vi "Read Channel info.vi"(8 "error in":errorcluster, 11 "channel in":refnum<class "StepNode.lvclass">) -> (0 "error out":errorcluster, 2 "channel info":T1, 3 "channel out":refnum<class "StepNode.lvclass">)   [LabVIEW 2015]
doc: "Copyright 2017 National Instruments Corporation\n\nLicensed under the Apache License, Version 2.0 (the \"License\"); you may not use this file except in compliance with the License. You may obtain a copy of the License at http://www.apache.org/licenses/LICENSE-2.0\nUnless required by applicable law or agreed to in writing, software distributed under the License is distributed on an \"AS IS\" BASIS, WITHOUT WARRANTIES OR CONDITIONS OF ANY KIND, either express or implied. See the License for the specific language governing permissions and limitations under the License."
uses:
  StepNode.lvclass
  to delete/ChannelData.ctl
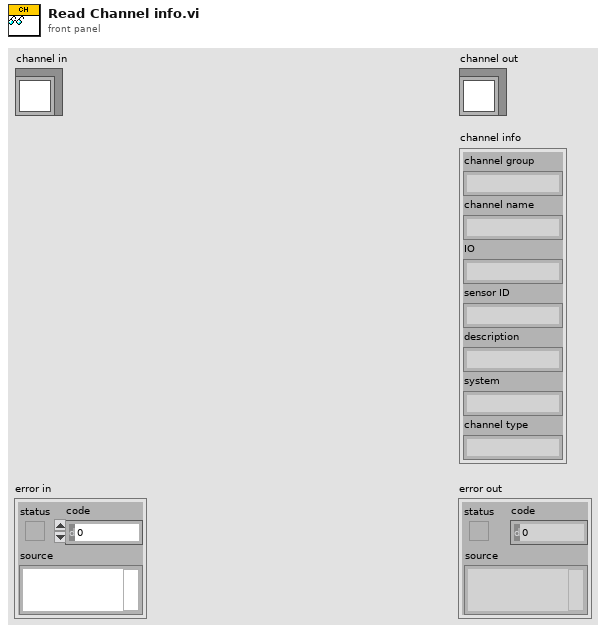
[diagram p1: front panel]
types:
  T1 = typedef "SequenceRepo.lvclass/ChannelData.ctl" = cluster{"channel group":string, "channel name":string, "IO ":string, "sensor ID":string, "description":string, "system":string, "channel type":string}
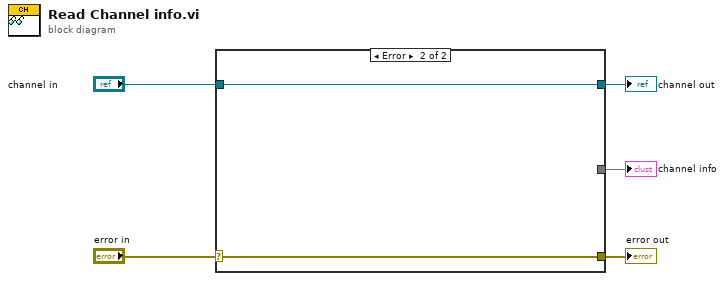
[diagram p0: block diagram]
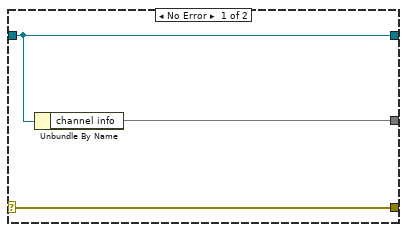
[diagram p2: hidden frame]
diagram:
  n1 = case shown="Error" "error in" {
    selector: "error in" -> [w8 w9]
    tunnel: [w8 w9] -> w4
    tunnel: [w7 w10] -> w2
    tunnel: "channel in" -> [w7 w10]
    tunnel: [w6 _] -> w1
    frame No Error {
      n2 = Unbundle By Name(w7) -> ("channel info"=w6)
    }
    frame Error {
    }
  }
  "error out" <- w4
  "channel out" <- w2
  "channel info" <- w1
